vi "insert alarmMap.vi"(0 "alarmMap":T1[](array[typedef]), 5 "error in (no error)":errorcluster) -> (19 "error out":errorcluster)   [LabVIEW 2016, in "opSignIn.lvlib"]
uses:
  opSignIn.lvlib
  alarmMap.ctl
  <vilib>/Utility/VariantDataType/VariantType.lvlib
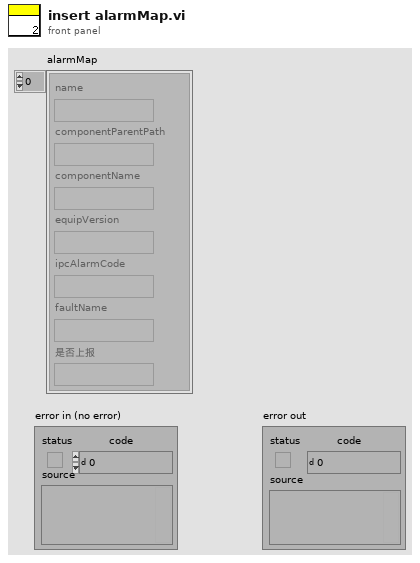
[diagram p1: front panel]
types:
  T1 = typedef "opSignIn.lvlib/alarmMap.ctl" = cluster{"name":string, "componentParentPath":string, "componentName":string, "equipVersion":string, "ipcAlarmCode":string, "faultName":string, "是否上报":string}
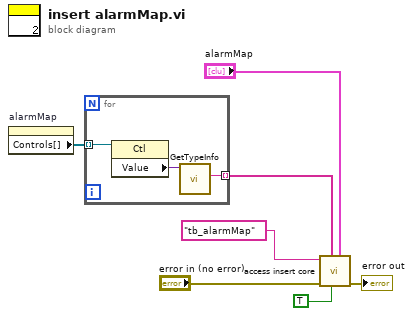
[diagram p0: block diagram]
diagram:
  n1 = property on="alarmMap" class="Clust (严格)"() -> ("Controls[]"=w7:refnum<vi>[])  [unwired: 2 in, 2 out]
  n2 = for {
    tunnel: w7 -> [w9] mode=indexing
    tunnel: [w10] -> w6 mode=indexing
    n3 = property class="Ctl"(reference=w9) -> ("Value"=w8:variant)  [unwired: 1 in, 2 out]
    n4 = call <vilib>:"GetTypeInfo.vi"("Variant"=w8) -> ("Name"=w10:string)  [unwired: 6 in, 4 out]
  }
  n5 = call "access insert core.vi"("data"="alarmMap", "delete table?"=TRUE, "columns"=w6, "error in (no error)"="error in (no error)", "table"="tb_alarmMap") -> ("error out"=→"error out":errorcluster)  [unwired: 6 in]
